vi "Read shared variable.vi"(10 "nome shared variable":string) -> (0 "error out":errorcluster, 2 "lettura":variant)   [LabVIEW 2019]
uses:
  Global IP address server.vi
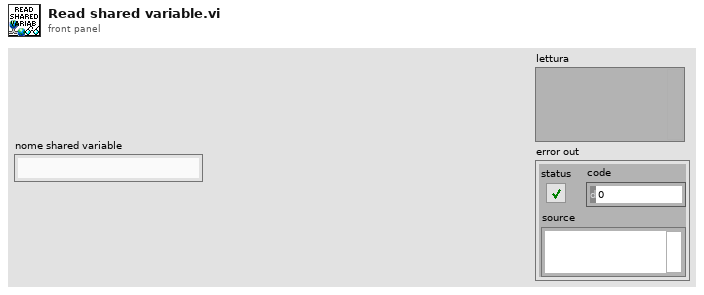
[diagram p1: front panel]
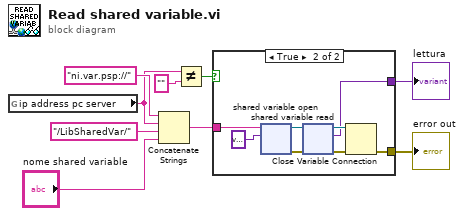
[diagram p0: block diagram]
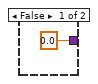
[diagram p2: hidden frame]
diagram:
  n1 = global read "Global IP address server.vi" "ip address pc server"() -> (w3:string)
  n2 = Concatenate Strings("ni.var.psp://", w3, "/LibSharedVar/", "nome shared variable") -> (w9:string)
  n3 = Not Equal?(x=w3, y="") -> (x != y?=w1:bool)
  n4 = case shown="True" w1 {
    tunnel: w9 -> [_ w18]
    tunnel: [0.0 w12] -> w5
    tunnel: [_ w11] -> w4
    frame False {
    }
    frame True {
      n5 = shared-variable-open(w18, variant) -> (w16:refnum<k21>, w17:errorcluster)  [unwired: 2 in]
      n6 = shared-variable-read(w16, w17) -> (w15:refnum<k21>, w14:errorcluster, w12:variant)  [unwired: 1 out]
      n7 = Close Variable Connection(8:w14, 11:w15) -> (0:w11:errorcluster)
    }
  }
  "lettura" <- w5
  "error out" <- w4
